vi "Key Press.vi"(8 "error in (no error)":errorcluster, 9 "ms wait after up (20)":u32=20, 10 "ms wait after down (80)":u32=80, 11 "Virtual Key":u8(ring)=65) -> (0 "error out":errorcluster)   [LabVIEW 2020, in "MacroAssert.lvlib"]
uses:
  MacroAssert.lvlib
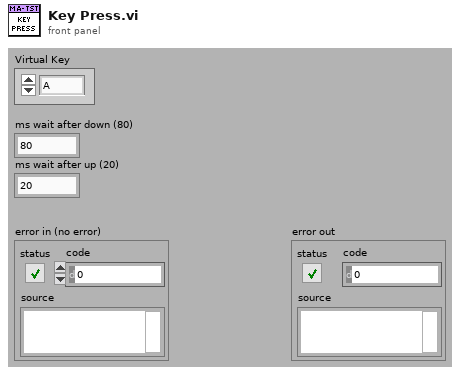
[diagram p1: front panel]
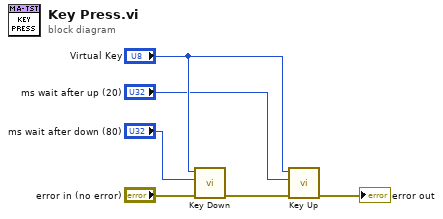
[diagram p0: block diagram]
diagram:
  n1 = call "Key Down.vi"("error in (no error)"="error in (no error)", "delay in ms (80)"="ms wait after down (80)", "Virtual Key"="Virtual Key") -> ("error out"=w4:errorcluster)  [unwired: 8 in]
  n2 = call "Key Up.vi"("error in (no error)"=w4, "delay in ms (20)"="ms wait after up (20)", "Virtual Key"="Virtual Key") -> ("error out"=→"error out":errorcluster)  [unwired: 8 in]
